vi "30_UNDT_Encoder2BInv (SubVI).vi"(8 "error in":errorcluster, 10 "Log":refnum<vi>, 11 "Encoder2BInv":bool) -> (0 "error out":errorcluster, 3 "Encoder2BInv_out":bool)   [LabVIEW 2017]
uses:
  Global_SNK3_HF.vi
  LV_Unicorn/LV_Unicorn.lvlib
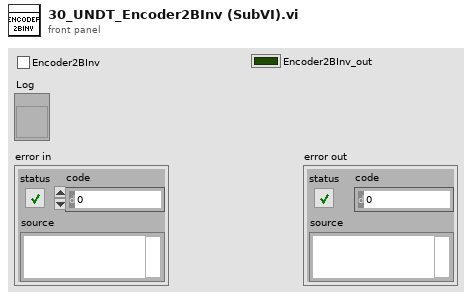
[diagram p1: front panel]
types:
  T1 = typedef "LV_Unicorn.lvlib/unicorn_Param.ctl" = cluster{"conParam":T2, "Param":T3}
  T2 = typedef "LV_Unicorn.lvlib/unicorn_conn.ctl" = cluster{"ReadIntParam":bool, "ReadDescrParam":bool, "ReadFloatParam":bool, "debug":bool, "ReadJSON":bool, "IP_address":string, "N_attempts":i32, "type_con":enum16{"Serial", "TCP"}, "MB_address":i32, "VISA":refnum<visa-resource-name>, "connection ID":refnum<k5>, "nameDevices":string, "timeout":i32, "port":u16, "type_version":string, "baud_rate":u32, "VersionControl":bool, "TCP_conn":bool, "WindowSize":i32}
  T3 = typedef "LV_Unicorn.lvlib/unicorn_JSON.ctl" = cluster{"NumParam":cluster{"NTelem":i32, "NInt":i32, "NFloat":i32, "NTable":i32}, "ParamInt":T4, "Telemetry":T5, "Table":T6, "ParamFloat":T7}
  T4 = typedef "LV_Unicorn.lvlib/unicorn_ParamInt.ctl" = cluster{"ID":string, "Num":i32, "Name":string, "Type":string, "Enum":string, "Desc":string, "Unit":string, "Access":string, "FormatStr":string, "Min":i32, "Max":i32}[]
  T5 = typedef "LV_Unicorn.lvlib/unicorn_Telemetry.ctl" = cluster{"ID":string, "Num":i32, "Name":string, "Desc":string, "Unit":string, "FormatStr":string, "Min":i32, "Max":i32}[]
  T6 = typedef "LV_Unicorn.lvlib/unicorn_Table.ctl" = cluster{"Num":i32, "Access":string, "ColumnCount":i32, "NeedParamPrepare":bool, "Columns":cluster{"Column":i32, "Desc":string, "Name":string}[], "DataType":string, "FormatStr":string, "ID":string, "Name":string, "RowCount":i32, "Rows":cluster{"Desc":string, "ID":string, "Max":i32, "Min":i32, "Name":string, "Row":i32, "Unit":string}[], "Type":string}[]
  T7 = typedef "LV_Unicorn.lvlib/unicorn_ParamFloat.ctl" = cluster{"ID":string, "Num":i32, "Name":string, "Type":string, "Enum":string, "Desc":string, "Unit":string, "Access":string, "FormatStr":string, "Min":sgl, "Max":sgl}[]
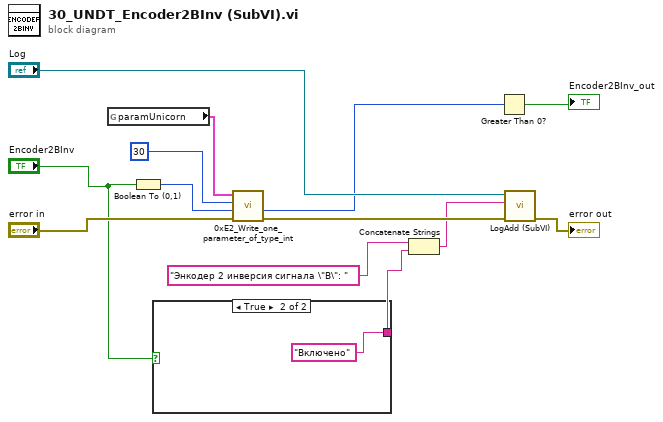
[diagram p0: block diagram]
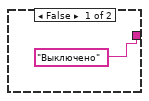
[diagram p2: hidden frame]
diagram:
  n1 = global read "Global_SNK3_HF.vi" "paramUnicorn"() -> (w12:T1)
  n2 = Boolean To (0,1)(Boolean="Encoder2BInv") -> (0, 1=w11:i16)
  n3 = case shown="True" "Encoder2BInv" {
    tunnel: ["Выключено" ("string") "Включено" ("string")] -> w2
    frame False {
    }
    frame True {
    }
  }
  n4 = call "0xE2_Write_one_parameter_of_type_int.vi"("error in"="error in", "ParamIn"=w11, "NumParamIn"=30 ("Номер параметра"), "paramUnicorn 2"=w12) -> ("error out"=w8:errorcluster, "ParamOut"=w5:i32)  [unwired: 4 in, 2 out]
  n5 = Concatenate Strings("Энкодер 2 инверсия сигнала \"B\": " ("string"), w2) -> (w1:string)
  n6 = Greater Than 0?(x=w5) -> (x > 0?=→"Encoder2BInv_out":bool)
  n7 = call "LogAdd (SubVI).vi"("error in"=w8, "string"=w1, "Log"="Log") -> ("error out"=→"error out":errorcluster)  [unwired: 8 in]
